vi "Initialise Spectrum Reader.vi"(8 "error in (no error)":errorcluster, 11 "IP Address":string) -> (0 "error out":errorcluster={"status"=TRUE, "code"=-314004, "source"="Create Network Stream Reader Endpoint in Initialise Spectrum Reader.vi->Host_Main.vi"}, 3 "Spectrum Reader":refnum<k21>)   [LabVIEW 2017]
doc: "Initialises the spectrum reader."
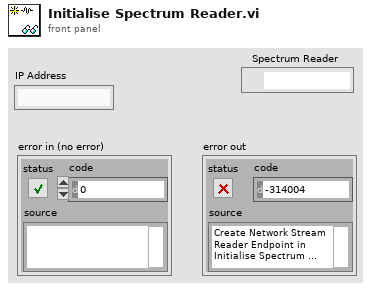
[diagram p1: front panel]
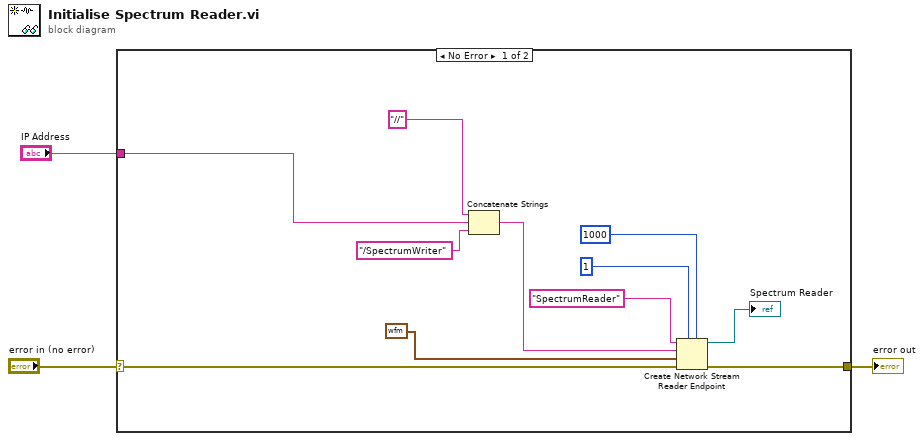
[diagram p0: block diagram]
diagram:
  n1 = case shown="No Error" "error in (no error)" {
    selector: "error in (no error)" -> [w7 w15]
    tunnel: [w13 w15] -> w3
    tunnel: "IP Address" -> [w4 _]
    frame No Error {
      n2 = Concatenate Strings("//", w4, "/SpectrumWriter" ("string")) -> (w8:string)
      n3 = Create Network Stream Reader Endpoint(5:1000 ("timeout in ms (-1)"), 7:1 ("reader buffer size"), 8:w7, 9:waveform(dbl) {"t0"=timestamp(0 s since 1904-01-01), "dt"=1.0, "Y"=[]} ("output waveform"), 10:w8, 11:"SpectrumReader" ("reader name")) -> (0:w13:errorcluster, 3:→"Spectrum Reader":refnum<k21>)  [unwired: 1 in]
    }
    frame Error {
    }
  }
  "error out" <- w3
